vi "PPCS_TRAJ_BEGIN.vi"(9 "Initial Gyo Reading":T3 {"SIN" format="%13.4f"; "COS" format="%13.4f"; "VALUE" format="%13.4f"}, 10 "Robot Starting Pose":T1 {"ROTATION"."SIN" format="%13.4f"; "ROTATION"."COS" format="%13.4f"; "ROTATION"."VALUE" format="%13.4f"; "TRANSLATION"."Y" format="%14.3f"; "TRANSLATION"."X" format="%14.3f"}) -> ()   [LabVIEW 2019]
uses:
  PPCS_TRAJECTORY_GLOBALS.vi
  <vilib>/Rock Robotics/WPI/ThirdParty/MJansen/PathPlanner/PathPlanner24.lvlib
  <vilib>/Rock Robotics/WPI/ThirdParty/JAS_Junk/TrajLib/TypeDef/TRANSLATION2D.ctl
  <vilib>/Rock Robotics/WPI/ThirdParty/JAS_Junk/TrajLib/Trajectory_Library.lvlib
  <vilib>/Rock Robotics/WPI/ThirdParty/JAS_Junk/TrajLib/TypeDef/ROTATION2D.ctl
  <vilib>/Rock Robotics/WPI/ThirdParty/JAS_Junk/TrajLib/TypeDef/POSE2D.ctl
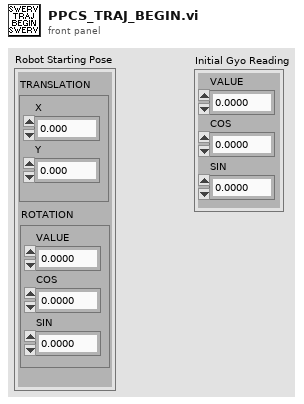
[diagram p1: front panel]
types:
  T1 = typedef "Trajectory_Library.lvlib/POSE2D.ctl" = cluster{"TRANSLATION":T2, "ROTATION":T3}
  T2 = typedef "Trajectory_Library.lvlib/TRANSLATION2D.ctl" = cluster{"X":dbl, "Y":dbl}
  T3 = typedef "Trajectory_Library.lvlib/ROTATION2D.ctl" = cluster{"VALUE":dbl, "COS":dbl, "SIN":dbl}
  T4 = typedef "PathPlanner24.lvlib/PathPlannerPath.ctl" = cluster{"BezierPoints":T2[], "PreviewStartingRotation":T3, "Reversed":bool, "RotationTargets":T5[], "ConstraintZones":T6[], "EventMarkers":T8[], "GlobalConstraints":T7, "GoalEndState":T11, "AllPoints":T12[]}
  T5 = typedef "PathPlanner24.lvlib/PathPlannerRotationTarget.ctl" = cluster{"target":T3, "WaypointRelativePosition":dbl, "Exists":bool}
  T6 = typedef "PathPlanner24.lvlib/PathPlannerConstraintsZone.ctl" = cluster{"minWaypointPos":dbl, "maxWaypointPos":dbl, "Constraints":T7, "Present":bool}
  T7 = typedef "PathPlanner24.lvlib/PathPlannerPathConstraints.ctl" = cluster{"MaxVelocityMps;":dbl, "MaxAccelerationMpsSq;":dbl, "MaxAngularVelRadPsEc;":dbl, "MaxAngularAccRadPSecSq":dbl, "Exists":bool}
  T8 = typedef "PathPlanner24.lvlib/PathPlannerEventMarker.ctl" = cluster{"WaypointRelativePos":dbl, "minimumTriggerDistance":dbl, "markerPos":T2, "lastRobotPos":T2, "Command":T9, "markerPos Exists":bool, "LastRobotPoseExists":bool, "Triggered":bool}
  T9 = typedef "PathPlanner24.lvlib/PathPlannerCommandUtil.ctl" = cluster{"waitTime":dbl, "name":string, "pathName":string, "commands":cluster{"type":T10, "waitTime":dbl, "name":string, "pathName":string}[], "type":T10}
  T10 = typedef "PathPlanner24.lvlib/PathPlanner_CommandUtilType_ENUM.ctl" = enum16{"Unknown", "Wait", "Named", "Path", "Sequential", "Parallel", "Race", "Deadline"}
  T11 = typedef "PathPlanner24.lvlib/PathPlannerGoalEndState.ctl" = cluster{"Velocity":dbl, "Rotation":T3}
  T12 = typedef "PathPlanner24.lvlib/PathPlannerPathPoint.ctl" = cluster{"Position":T2, "HolonomicRotation":T3, "DistAlongPath":dbl, "CurveRadius":dbl, "MaxV":dbl, "Constraints":T7, "HolonomicRotationExists":bool}
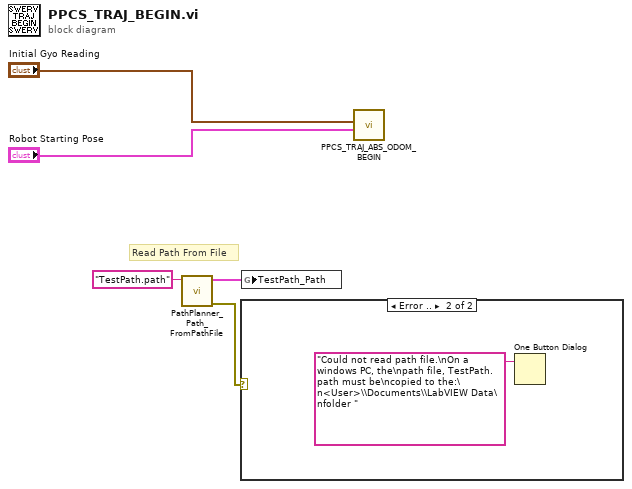
[diagram p0: block diagram]
diagram:
  # "Read Path From File"
  n1 = call <vilib>:"PathPlanner_Path_FromPathFile.vi"("FileName"="TestPath.path") -> ("error out"=w1:errorcluster, "PathPlannerPath"=w2:T4)  [unwired: 8 in, 1 out]
  n2 = case shown="Error .." w1 {
    frame No Error {
    }
    frame Error {
      n3 = One Button Dialog(message="Could not read path file.\nOn a windows PC, the\npath file, TestPath.path must be\ncopied to the:\n<User>\\Documents\\LabVIEW Data\nfolder ") -> ()  [unwired: 1 in, 1 out]
    }
  }
  n4 = global write "PPCS_TRAJECTORY_GLOBALS.vi" "TestPath_Path"(w2) -> ()
  n5 = call "PPCS_TRAJ_ABS_ODOM_BEGIN.vi"("Initial Pose"="Robot Starting Pose", "Initial Gyro Angle"="Initial Gyo Reading") -> ()  [unwired: 9 in, 1 out]
